vi "Actor Core.vi"(8 "error in":errorcluster, 11 "ServerListener in":refnum<class "ServerListener.lvclass">) -> (0 "error out":errorcluster, 3 "Actor out":refnum<class "Actor.lvclass">)   [LabVIEW 2013, in "ServerListener.lvlib" / "ServerListener.lvclass"]
doc: "(<B>Filename</B>: Actor Framework.lvlib:Actor.lvclass:Actor Core.vi)\n\nReceives messages to the actor, reacts to them, and initiates any error handling that may shut the actor down.\n\nDescendant classes may override this VI to append parallel tasks for the actor to complete while it handles messages. Overrides use the Call Parent Method node."
uses:
  ServerListener.lvclass
  <vilib>/ActorFramework/Actor/Actor.lvclass
  <vilib>/ActorFramework/Actor/Actor.lvclass/Actor.ctl
  <vilib>/ActorFramework/Message Enqueuer/Message Enqueuer.lvclass/Message Enqueuer.ctl
  Add Connection Msg/Add Connection Msg.lvclass/Add Connection Msg.ctl
  <vilib>/ActorFramework/Message Enqueuer/Init from Existing Queue.vi
  <vilib>/ActorFramework/Message Enqueuer/Enqueue.vi
  <vilib>/ActorFramework/Message Priority Queue/Priority Enqueue.vi
  <vilib>/ActorFramework/Message Enqueuer/Message Enqueuer.lvclass
  Add Connection Msg/Add Connection Msg.lvclass
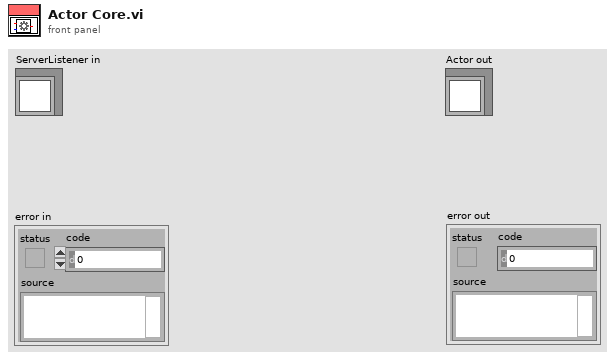
[diagram p1: front panel]
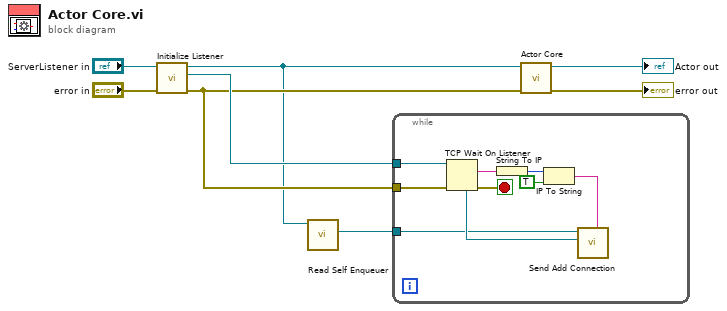
[diagram p0: block diagram]
diagram:
  n1 = call "Initialize Listener.vi"("error in (no error)"="error in", "ServerListener in"="ServerListener in") -> ("error out"=w2:errorcluster, "listener ID"=w3:refnum<k5>, "ServerListener out"=w1:refnum<class "ServerListener.lvclass">)  [unwired: 7 in]
  n2 = call <vilib>:"Read Self Enqueuer.vi"("Actor"=w1) -> ("Self Enqueuer"=w6:refnum<class "Message Enqueuer.lvclass">)  [unwired: 10 in]
  n3 = while {
    tunnel: w3 -> [w17]
    tunnel: w2 -> [w16]
    tunnel: w6 -> [w13]
    stop <- w15 stop-if-true
    n4 = TCP Wait On Listener(8:w16, 11:w17) -> (0:w15:errorcluster, 2:w12:string, 4:w14:refnum<k5>)  [unwired: 2 in, 2 out]
    n5 = String To IP(1:w12) -> (0:w11:u32)
    n6 = IP To String(1:TRUE ("dot notation? (F)"), 2:w11) -> (0:w9:string)
    n7 = call "Send Add Connection.vi"("remote address"=w9, "connection ID"=w14, "Message Enqueuer"=w13) -> ()  [unwired: 7 in, 2 out]
  }
  n8 = call-parent "Actor Core.vi"("error in"=w2, "Actor in"=w1) -> ("error out"=→"error out":errorcluster, "Actor out"=→"Actor out":refnum<class "Actor.lvclass">)  [unwired: 8 in]
